vi "Generate Static Image.vi"(8 "error in (no error)":errorcluster, 10 "Image Y Size":i32, 11 "Image X Size":i32) -> (0 "error out":errorcluster, 3 "Image 2":T2(plugin-control))   [LabVIEW 2012]
doc: "SciScan 1.2 160622"
uses:
  <vilib>/vision/NI_Vision_Development_Module.lvlib
panel:
  out "Image Type":T1 items=["Grayscale (U8)", "Grayscale (I16)", "Grayscale (SGL)", "Complex (CSG)", "RGB (U32)", "HSL (U32)", "RGB (U64)", "Grayscale (U16)"]
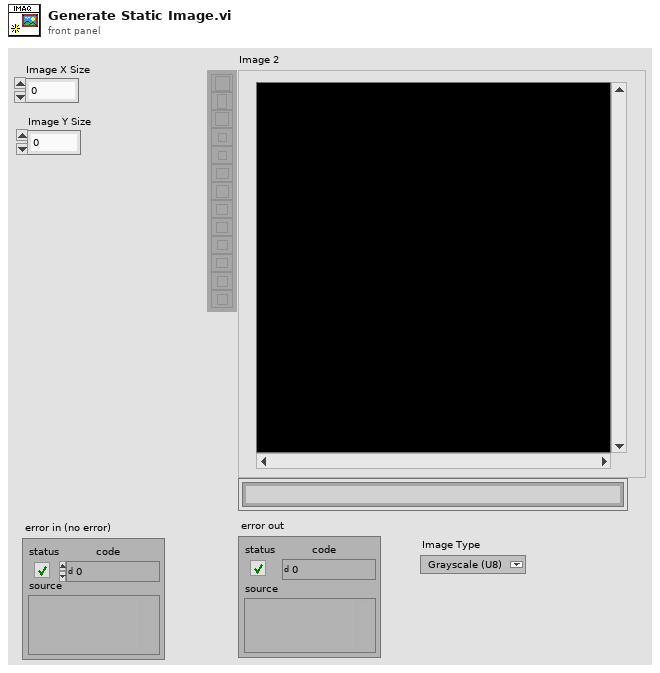
[diagram p1: front panel]
types:
  T1 = typedef "Image Type" = u32
  T2 = typedef "IMAQ Image.ctl" = refnum<image>
  T3 = cluster{"Read Raw File":i32, "File Data Type":u32, "Offset to Data":i32, "Use Min Max":enum32{"Don't use min max", "Use file values", "Use optional values"}, "Optional Min Value":sgl, "Optional Max Value":sgl, "Byte Order":enum32{"Big endian (Motorola)", "Little endian (Intel)"}}
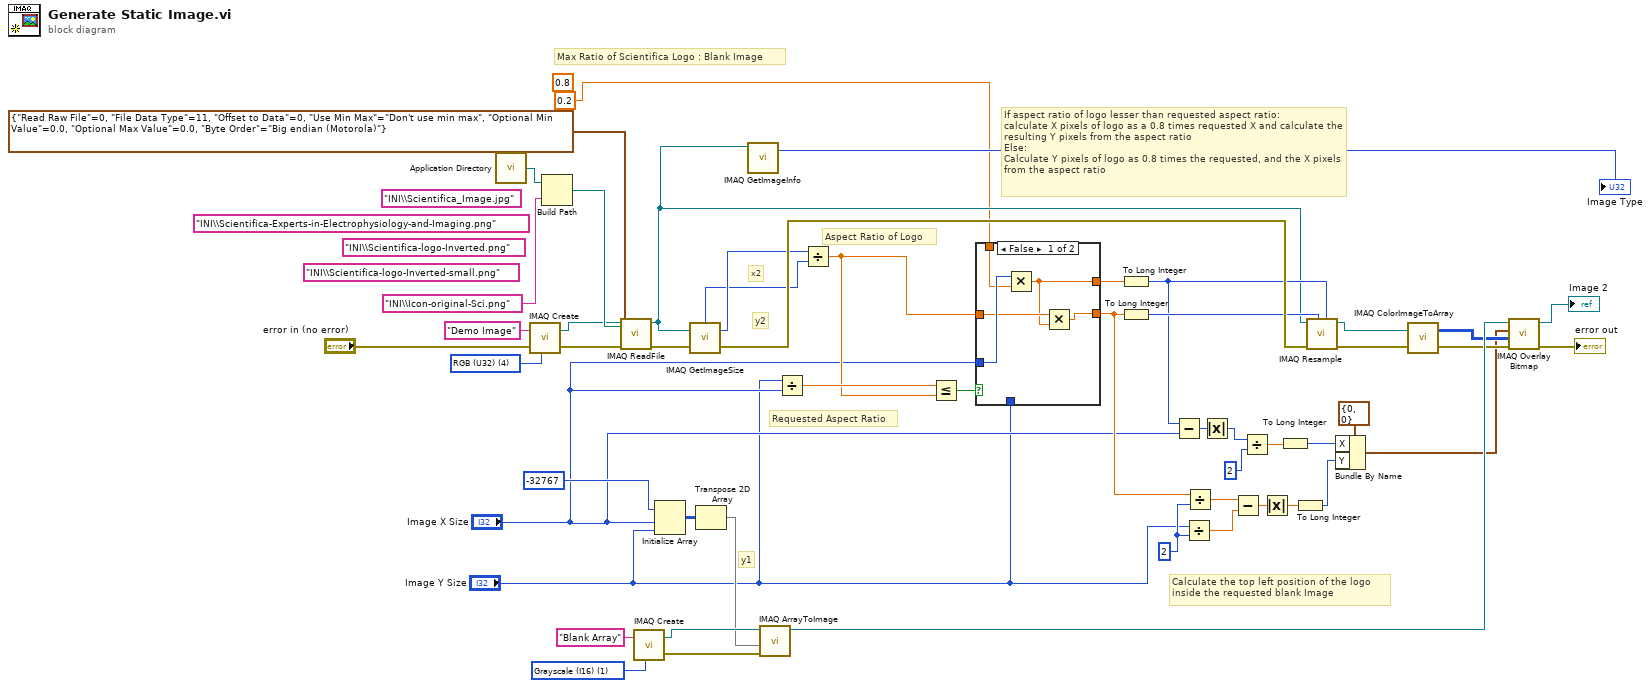
[diagram p0: block diagram]
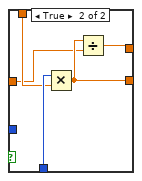
[diagram p2: hidden frame]
diagram:
  (unwired) "INI\\Scientifica-logo-Inverted-small.png" ("name or relative path")
  w17 = 2 ("y")
  (unwired) 0.8 ("y")
  w40 = T1 4 items=["Grayscale (U8)", "Grayscale (I16)", "Grayscale (SGL)", "Complex (CSG)", "RGB (U32)", "HSL (U32)", "RGB (U64)", "Grayscale (U16)"] ("Image Type")
  w45 = T1 1 items=["Grayscale (U8)", "Grayscale (I16)", "Grayscale (SGL)", "Complex (CSG)", "RGB (U32)", "HSL (U32)", "RGB (U64)", "Grayscale (U16)"] ("Image Type")
  (unwired) "INI\\Scientifica-logo-Inverted.png" ("name or relative path")
  (unwired) "INI\\Scientifica-Experts-in-Electrophysiology-and-Imaging.png" ("name or relative path")
  (unwired) "INI\\Scientifica_Image.jpg" ("name or relative path")
  # "Calculate the top left position of the logo\ninside the requested blank Image"
  # "If aspect ratio of logo lesser than requested aspect ratio:\ncalculate X pixels of logo as a 0.8 times requested X and calculate the resulting Y pixels from the aspect ratio\nElse:\nCalculate Y pixels of logo as 0.8 times the requested, and the X pixels from the aspect ratio"
  # "Requested Aspect Ratio"
  # "Max Ratio of Scientifica Logo : Blank Image"
  # "Aspect Ratio of Logo"
  # "y2"
  # "x2"
  # "y1"
  n1 = call <vilib>:"Application Directory.vi"() -> ("Application Directory"=w52:path)
  n2 = call "IMAQ Create"("Image Name"="Demo Image", "Image Type"=w40, "error in (no error)"="error in (no error)") -> ("New Image"=w43:T2, "error out"=w42:errorcluster)  [unwired: 2 in]
  n3 = Build Path(base path=w52, name or relative path="INI\\Icon-original-Sci.png") -> (appended path=w46:path)
  n4 = call "IMAQ ReadFile"("File Path"=w46, "error in (no error)"=w42, "File Options"=T3 {"Read Raw File"=0, "File Data Type"=11, "Offset to Data"=0, "Use Min Max"=enum."Don't use min max", "Optional Min Value"=0.0, "Optional Max Value"=0.0, "Byte Order"=enum."Big endian (Motorola)"}, "Image"=w43) -> ("error out"=w36:errorcluster, "Image Out"=w3:T2)  [unwired: 3 in, 3 out]
  n5 = call "IMAQ Create"("Image Name"="Blank Array", "Image Type"=w45) -> ("New Image"=w48:T2, "error out"=w37:errorcluster)  [unwired: 3 in]
  n6 = Initialize Array(i16 -32767, "Image X Size", "Image Y Size") -> (w22:i16[][])
  n7 = call "IMAQ GetImageSize"("Image"=w3, "error in (no error)"=w36) -> ("Y Resolution"=w24:i32, "X Resolution"=w23:i32, "error out"=w35:errorcluster)  [unwired: 2 in]
  n8 = Transpose 2D Array(2D array=w22) -> (transposed array=w21:i16[][])
  n9 = call "IMAQ GetImageInfo"("Image"=w3) -> ("Image Type"=→"Image Type":T1)  [unwired: 3 in, 7 out]
  n10 = call "IMAQ ArrayToImage"("error in (no error)"=w37, "Image Pixels (I16)"=w21, "Image"=w48) -> ("Image Out"=w47:T2)  [unwired: 7 in, 1 out]
  n11 = Divide(x="Image Y Size", y="Image X Size") -> (x/y=w12:dbl)
  n12 = Divide(x=w24, y=w23) -> (x/y=w11:dbl)
  n13 = Less Or Equal?(x=w12, y=w11) -> (x <= y?=w13:bool)
  n14 = case shown="False" w13 {
    tunnel: "Image X Size" -> [w57 _]
    tunnel: 0.2 ("y") -> [w56 w61]
    tunnel: [w54 w60] -> w9
    tunnel: w11 -> [w55 w58]
    tunnel: [w53 w59] -> w10
    tunnel: "Image Y Size" -> [_ w62]
    frame False {
      n15 = Multiply(x=w57, y=w56) -> (x*y=w54:dbl)
      n16 = Multiply(x=w55, y=w54) -> (x*y=w53:dbl)
    }
    frame True {
      n17 = Multiply(x=w62, y=w61) -> (x*y=w59:dbl)
      n18 = Divide(x=w59, y=w58) -> (x/y=w60:dbl)
    }
  }
  n19 = To Long Integer(number=w9) -> (32bit integer=w14:i32)
  n20 = To Long Integer(number=w10) -> (32bit integer=w15:i32)
  n21 = Subtract(x=w14, y="Image X Size") -> (x-y=w31:i32)
  n22 = Divide(x="Image Y Size", y=w17) -> (x/y=w18:dbl)
  n23 = Divide(x=w10, y=w17) -> (x/y=w16:dbl)
  n24 = Absolute Value(x=w31) -> (abs(x)=w30:i32)
  n25 = Subtract(x=w16, y=w18) -> (x-y=w20:dbl)
  n26 = Divide(x=w30, y=2) -> (x/y=w28:dbl)
  n27 = Absolute Value(x=w20) -> (abs(x)=w19:dbl)
  n28 = To Long Integer(number=w28) -> (32bit integer=w27:i32)
  n29 = To Long Integer(number=w19) -> (32bit integer=w26:i32)
  n30 = call "IMAQ Resample"("X Resolution"=w14, "Y Resolution"=w15, "error in (no error)"=w35, "Image Src"=w3) -> ("error out"=w33:errorcluster, "Image Dst Out"=w34:T2)  [unwired: 6 in]
  n31 = Bundle By Name(cluster=cluster{"X":i32, "Y":i32} {"X"=0, "Y"=0} ("Top Left Point"), "X"=w27, "Y"=w26) -> (w25:cluster{"X":i32, "Y":i32})
  n32 = call "IMAQ ColorImageToArray"("Image"=w34, "error in (no error)"=w33) -> ("Image Pixels (U32)"=w39:u32[][], "error out"=w38:errorcluster)  [unwired: 2 in, 1 out]
  n33 = call "IMAQ Overlay Bitmap"("error in (no error)"=w38, "Bitmap"=w39, "Top Left Point"=w25, "Image"=w47) -> ("error out"=→"error out":errorcluster, "Image Out"=→"Image 2":T2)  [unwired: 6 in]
